vi "SendSfxUL_Addon.vi"(6 "Resp Timeout (ms)":i32=1000 min=0, 7 "Active Dut":T1=enum."DUT 2", 8 "Error In":errorcluster, 9 "Test Mode":i8=1, 10 "Pwr Reduction (dB/2)":i8=1, 11 "FPGA Reference":refnum<k20>) -> (0 "Error Out":errorcluster, 1 "reduce resp":string="reduce_output_power -30\r\n{{(redu", 2 "Tx Testmode OK":bool, 3 "test_mode_resp":string, 4 "switch resp":string="switch_pa 1\r\n{{(switch_pa)} API ")   [LabVIEW 2018]
uses:
  Resources_Test/UART/ControlTestSlot.ctl
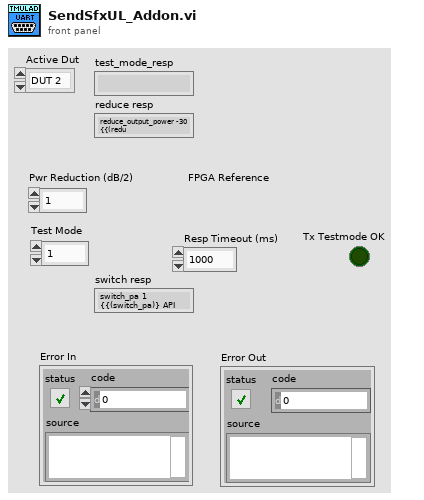
[diagram p1: front panel]
types:
  T1 = typedef "ControlTestSlot.ctl" = enum16{"DUT 1", "DUT 2"}
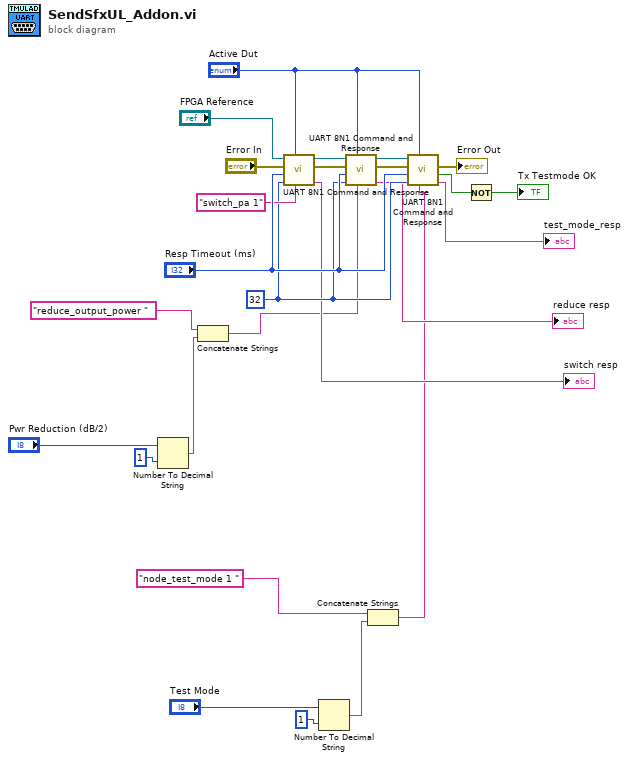
[diagram p0: block diagram]
diagram:
  w15 = u32 32 ("Response Size (char)")
  n1 = Number To Decimal String(number="Pwr Reduction (dB/2)", width (-)=i16 1) -> (decimal integer string=w6:string)
  n2 = Concatenate Strings("reduce_output_power " ("Text to Send"), w6) -> (w10:string)
  n3 = call "UART 8N1 Command and Response.vi"("Text to Send"="switch_pa 1", "Active Dut"="Active Dut", "Response Size (char)"=w15, "Response Timeout (ms)"="Resp Timeout (ms)", "Error In"="Error In", "FPGA VI Reference In"="FPGA Reference") -> ("Received Text"=→"switch resp":string, "Error Out"=w22:errorcluster, "FPGA VI Reference Out"=w21:refnum<k20>)  [unwired: 1 in, 2 out]
  n4 = Number To Decimal String(number="Test Mode", width (-)=i16 1) -> (decimal integer string=w3:string)
  n5 = call "UART 8N1 Command and Response.vi"("Text to Send"=w10, "Active Dut"="Active Dut", "Response Size (char)"=w15, "Response Timeout (ms)"="Resp Timeout (ms)", "Error In"=w22, "FPGA VI Reference In"=w21) -> ("Received Text"=→"reduce resp":string, "Error Out"=w18:errorcluster, "FPGA VI Reference Out"=w20:refnum<k20>)  [unwired: 1 in, 2 out]
  n6 = Concatenate Strings("node_test_mode 1 " ("Text to Send"), w3) -> (w1:string)
  n7 = call "UART 8N1 Command and Response.vi"("Text to Send"=w1, "Active Dut"="Active Dut", "Response Size (char)"=w15, "Response Timeout (ms)"="Resp Timeout (ms)", "Error In"=w18, "FPGA VI Reference In"=w20) -> ("Received Text"=→"test_mode_resp":string, "Timeout Flag"=w25:bool, "Error Out"=→"Error Out":errorcluster)  [unwired: 1 in, 2 out]
  n8 = Not(x=w25) -> (.not. x?=→"Tx Testmode OK":bool)
